vi "Uniform Moments.vi"(9 "xmax":dbl=1.0, 10 "xmin":dbl) -> (0 "error":i32, 2 "variance":dbl=1.0, 3 "mean":dbl)   [LabVIEW 2020, in "NI_Gmath.lvlib"]
doc: "Returns the expected mean and variance of the random variate X, where X describes the selected distribution type. You must manually select the polymorphic instance to use."
uses:
  NI_Gmath.lvlib
  st_error_code.ctl
panel:
  # "Uniform Moments"
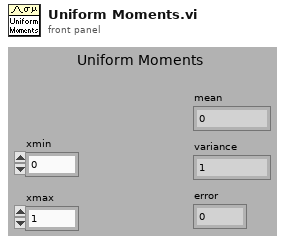
[diagram p1: front panel]
types:
  T1 = typedef "NI_Gmath.lvlib/st_error_code.ctl" = i32
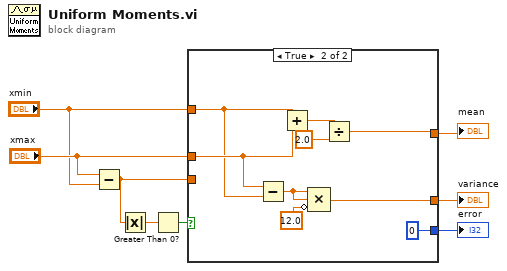
[diagram p0: block diagram]
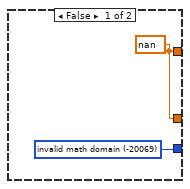
[diagram p2: hidden frame]
diagram:
  n1 = Subtract(x="xmax", y="xmin") -> (x-y=w5:dbl)
  n2 = Absolute Value(x=w5) -> (abs(x)=w6:dbl)
  n3 = Greater Than 0?(x=w6) -> (x > 0?=w4:bool)
  n4 = case shown="True" w4 {
    tunnel: "xmax" -> [_ w15]
    tunnel: "xmin" -> [_ w14]
    tunnel: w5 -> [_ _]
    tunnel: [w10 w16] -> w3
    tunnel: [w9 0] -> w2
    tunnel: [w10 w11] -> w1
    frame False {
      w9 = T1 -20069 items=["invalid math domain"=-20069, "Fourier interpolation size m >= n"=-20070, "empty array"=-20003] ("stat interp error code")
      w10 = nan
    }
    frame True {
      n5 = Subtract(x=w15, y=w14) -> (x-y=w13:dbl)
      n6 = Add(x=w14, y=w15) -> (x+y=w18:dbl)
      n7 = Compound Arithmetic op=MULTIPLY(w13, w13, invert 12.0 ("y")) -> (w11:dbl)
      n8 = Divide(x=w18, y=2.0) -> (x/y=w16:dbl)
    }
  }
  "mean" <- w3
  "error" <- w2
  "variance" <- w1
